vi "VerifyScannerReadOut.vi"(9 "IgnoreOCR":bool, 10 "ScanerReadOut":string[](array[string]), 11 "LaserVariables":string[](array[string])) -> (0 "WrongScannerRead":string, 1 "WrongLaserVar":string, 3 "Equal":bool)   [LabVIEW 2016]
uses:
  V7310/LowLevel/V7310.Global.vi
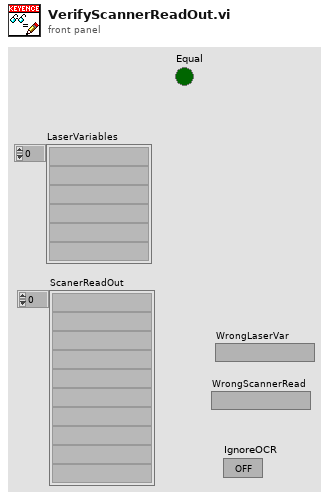
[diagram p1: front panel]
types:
  T1 = typedef "V7310.Data.Status.ctl" = cluster{"State":T2, "LaserStatus":T3, "LaserStatusRaw":string, "Ref":refnum<k5>, "RTC TS":timestamp, "Conn TS":timestamp, "Msg":T4[], "JobInUse":string, "Jobs":string[], "Vars":T5[]}
  T2 = typedef "V7310.Data.Status.State.ctl" = enum16{"First", "Init", "Msg", "Error", "Abort", "Idle", "Run"}
  T3 = typedef "V7310.LaserStatus.ctl" = enum16{"-", "FatalError", "Initialize", "KeySwitchOpen", "TimeoutInterlock", "InterlockOpen", "StartUp", "ShutterlockOpen", "Standby", "Ready", "PrepareForMarking", "WaitForTrigger", "Marking"}
  T4 = typedef "V7310.Message.Data.ctl" = cluster{"ID":i32, "Msg":string}
  T5 = typedef "V7310.Job.Variable.ctl" = cluster{"Name":string, "Value":string}
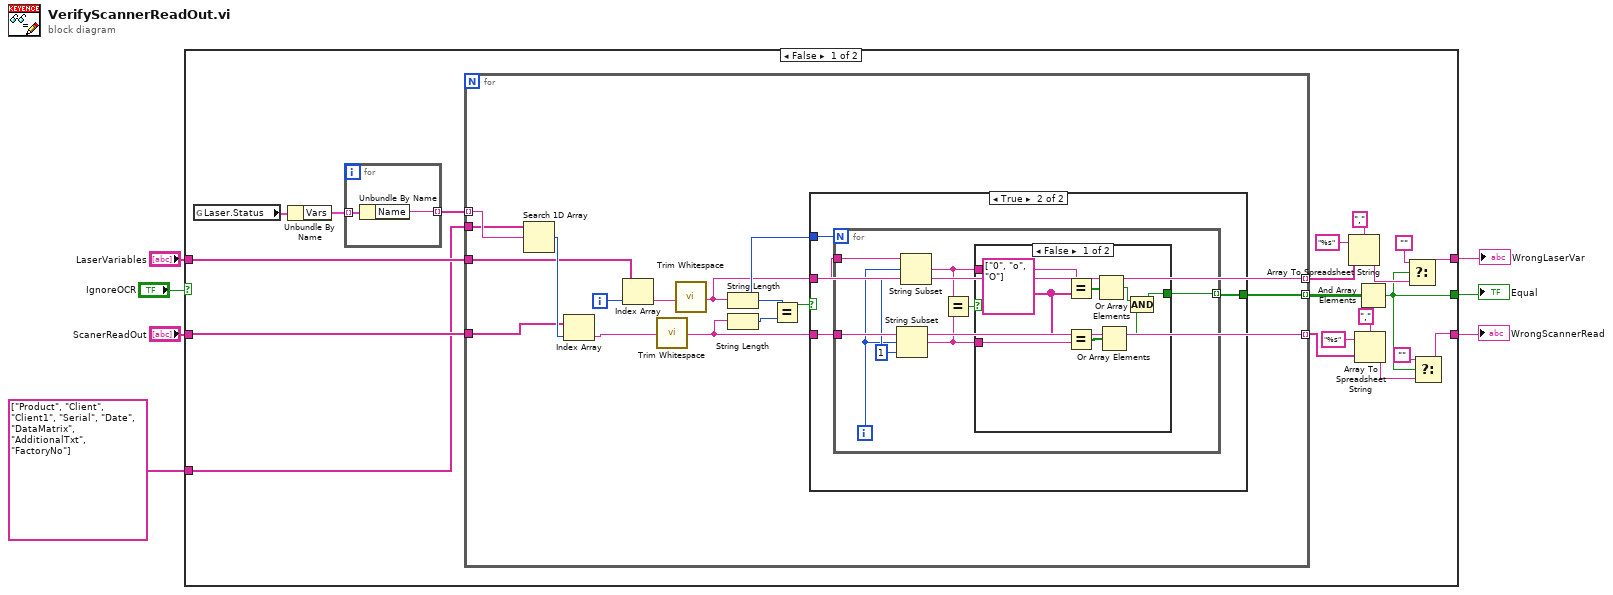
[diagram p0: block diagram]
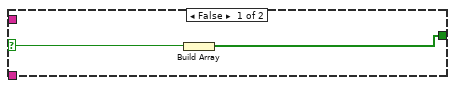
[diagram p2: hidden frame]
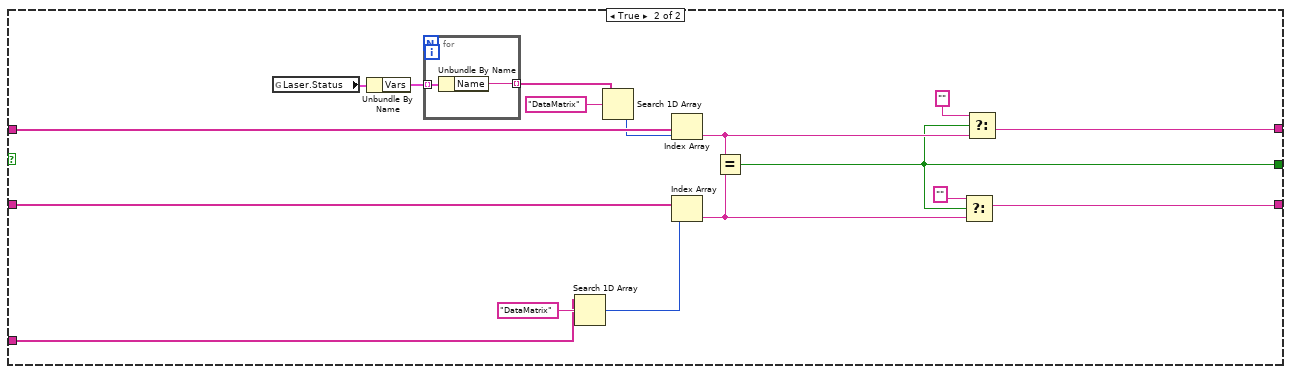
[diagram p4: hidden frame]
diagram:
  n1 = case shown="False" "IgnoreOCR" {
    tunnel: "LaserVariables" -> [w24 w79]
    tunnel: [w9 w69] -> w1
    tunnel: [w15 w67] -> w6
    tunnel: [w8 w68] -> w5
    tunnel: "ScanerReadOut" -> [w23 w78]
    tunnel: string[] ["Product", "Client", "Client1", "Serial", "Date", "DataMatrix", "AdditionalTxt", "FactoryNo"] -> [w22 w76]
    frame False {
      n2 = global read "V7310.Global.vi" "Laser.Status"() -> (w27:T1)
      n3 = Unbundle By Name(w27) -> ("Vars"=w26:T5[])
      n4 = for {
        tunnel: w26 -> [w66] mode=indexing
        tunnel: [w65] -> w25 mode=indexing
        n5 = Unbundle By Name(w66) -> ("Name"=w65:string)
      }
      n6 = for {
        tunnel: [w37] -> w21 mode=indexing
        tunnel: [w29] -> w11 mode=indexing
        tunnel: w25 -> [w41] mode=indexing
        tunnel: w22 -> [w40]
        tunnel: w24 -> [w36]
        tunnel: w23 -> [w38]
        tunnel: [w28] -> w20 mode=indexing
        i -> [w35]
        n7 = Search 1D Array(1D array=w40, element=w41) -> (index of element=w39:i32)  [unwired: 1 in]
        n8 = Index Array(array=w38, index=w39) -> (element=w32:string)
        n9 = Index Array(array=w36, index=w35) -> (element=w34:string)
        n10 = call <vilib>:"Trim Whitespace.vi"("string"=w32) -> ("trimmed string"=w29:string)  [unwired: 1 in]
        n11 = call <vilib>:"Trim Whitespace.vi"("string"=w34) -> ("trimmed string"=w28:string)  [unwired: 1 in]
        n12 = String Length(string=w28) -> (length=w31:i32)
        n13 = String Length(string=w29) -> (length=w33:i32)
        n14 = Equal?(x=w31, y=w33) -> (x = y?=w30:bool)
        n15 = case shown="True" w30 {
          selector: w30 -> [w43 _]
          tunnel: [w42 w45] -> w37
          tunnel: w29 -> [_ w47]
          tunnel: w31 -> [_ w46]
          tunnel: w28 -> [_ w44]
          frame False {
            n16 = Build Array(w43) -> (w42:bool[])
          }
          frame True {
            n17 = for {
              N: w46 -> [_]
              tunnel: w44 -> [w49]
              tunnel: w47 -> [w50]
              tunnel: [w48] -> w45 mode=indexing
              i -> [w54]
              w55 = 1 ("length (rest)")
              n18 = String Subset(string=w50, offset (0)=w54, length (rest)=w55) -> (substring=w51:string)
              n19 = String Subset(string=w49, offset (0)=w54, length (rest)=w55) -> (substring=w52:string)
              n20 = Equal?(x=w52, y=w51) -> (x = y?=w53:bool)
              n21 = case shown="False" w53 {
                selector: w53 -> [_ w64]
                tunnel: [w56 w64] -> w48
                tunnel: w52 -> [w63 _]
                tunnel: w51 -> [w61 _]
                frame False {
                  w60 = string[] ["0", "o", "O"]
                  n22 = Equal?(x=w63, y=w60) -> (x = y?=w62:bool[])
                  n23 = Equal?(x=w60, y=w61) -> (x = y?=w59:bool[])
                  n24 = Or Array Elements(Boolean array=w62) -> (logical OR=w58:bool)
                  n25 = Or Array Elements(Boolean array=w59) -> (logical OR=w57:bool)
                  n26 = Compound Arithmetic op=AND(w58, w57) -> (w56:bool)
                }
                frame True {
                }
              }
            }
          }
        }
      }
      n27 = Array To Spreadsheet String(delimiter (Tab)=",", array=w20, 3:"%s" ("format string")) -> (spreadsheet string=w17:string)
      n28 = Array To Spreadsheet String(delimiter (Tab)=",", array=w11, 3:"%s" ("format string")) -> (spreadsheet string=w10:string)
      n29 = And Array Elements(Boolean array=w21) -> (logical AND=w9:bool)
      n30 = Select(t="", s=w9, f=w17) -> (s? t:f=w15:string)
      n31 = Select(t="", s=w9, f=w10) -> (s? t:f=w8:string)
    }
    frame True {
      n32 = global read "V7310.Global.vi" "Laser.Status"() -> (w83:T1)
      n33 = Unbundle By Name(w83) -> ("Vars"=w82:T5[])
      n34 = for {
        tunnel: w82 -> [w85] mode=indexing
        tunnel: [w84] -> w81 mode=indexing
        n35 = Unbundle By Name(w85) -> ("Name"=w84:string)
      }
      n36 = Search 1D Array(1D array=w76, element="DataMatrix") -> (index of element=w75:i32)  [unwired: 1 in]
      n37 = Search 1D Array(1D array=w81, element="DataMatrix") -> (index of element=w74:i32)  [unwired: 1 in]
      n38 = Index Array(array=w79, index=w74) -> (element=w71:string)
      n39 = Index Array(array=w78, index=w75) -> (element=w70:string)
      n40 = Equal?(x=w71, y=w70) -> (x = y?=w69:bool)
      n41 = Select(t="", s=w69, f=w70) -> (s? t:f=w68:string)
      n42 = Select(t="", s=w69, f=w71) -> (s? t:f=w67:string)
    }
  }
  "Equal" <- w1
  "WrongLaserVar" <- w6
  "WrongScannerRead" <- w5
